vi "FABR-Init I-O Plot.vi"(0 "I-O":refnum<vi>, 5 "IOLegend":refnum<vi>, 7 "Freq":dbl[](array[numeric]), 9 "Level":dbl[](array[numeric]), 11 "error in (no error)":errorcluster) -> (15 "error out":errorcluster)   [LabVIEW 2020]
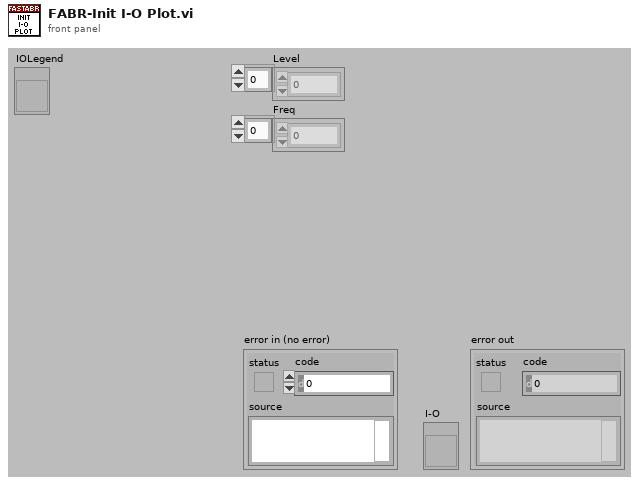
[diagram p1: front panel]
types:
  T1 = enum16{"User", "Prism", "Kelly", "Dark2", "Sequential", "Hue"}
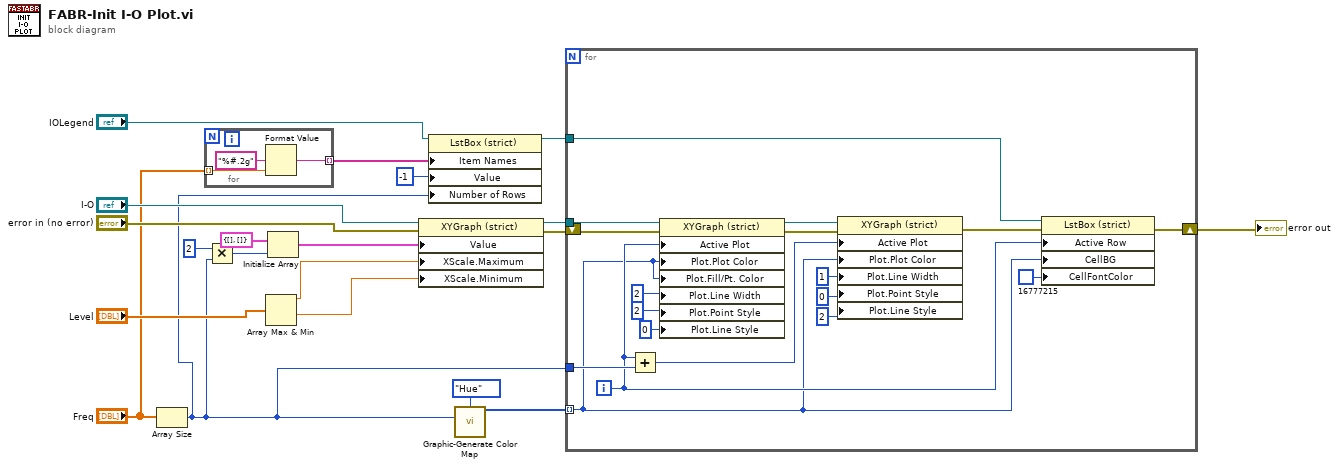
[diagram p0: block diagram]
diagram:
  n1 = Array Size(array="Freq") -> (size(s)=w1:i32)
  n2 = for {
    tunnel: "Freq" -> [w23] mode=indexing
    tunnel: [w21] -> w4 mode=indexing
    n3 = Format Value(format string="%#.2g", value (0)=w23) -> (output string=w21:string)  [unwired: 1 in]
  }
  n4 = Multiply(x=2, y=w1) -> (x*y=w12:i32)
  n5 = Array Max & Min(array="Level") -> (max value=w18:dbl, min value=w17:dbl)  [unwired: 2 out]
  n6 = Initialize Array(cluster{dbl[], dbl[]} {[], []}, w12) -> (w11:cluster{dbl[], dbl[]}[])
  n7 = property class="XYGraph (strict)"(reference="I-O", error in="error in (no error)", "Value"=w11, "XScale.Maximum"=w18, "XScale.Minimum"=w17) -> (reference out=w10:refnum<vi>, error out=w9:errorcluster)
  n8 = property class="LstBox (strict)"(reference="IOLegend", "Item Names"=w4, "Value"=-1 ("Focus Row"), "Number of Rows"=w1) -> (reference out=w3:refnum<vi>)  [unwired: 1 in, 1 out]
  n9 = call "Graphic-Generate Color Map.vi"("Map"=T1."Hue", "Size"=w1) -> ("Colors"=w8:u32[])  [unwired: 13 in]
  n10 = for {
    tunnel: w10 -> [w41]
    tunnel: w8 -> [w25] mode=indexing
    tunnel: w1 -> [w35]
    shift-right: [w27] -> w7
    shift-left: w9 -> [w40]
    tunnel: w3 -> [w29]
    i -> [w26]
    n11 = Add(x=w26, y=w35) -> (x+y=w34:i32)
    n12 = property class="XYGraph (strict)"(reference=w41, error in=w40, "Active Plot"=w26, "Plot.Plot Color"=w25, "Plot.Fill/Pt. Color"=w25, "Plot.Line Width"=u8 2, "Plot.Point Style"=u8 2, "Plot.Line Style"=u8 0) -> (reference out=w37:refnum<vi>, error out=w36:errorcluster)
    n13 = property class="XYGraph (strict)"(reference=w37, error in=w36, "Active Plot"=w34, "Plot.Plot Color"=w25, "Plot.Line Width"=u8 1, "Plot.Point Style"=u8 0, "Plot.Line Style"=u8 2) -> (error out=w28:errorcluster)  [unwired: 1 out]
    n14 = property class="LstBox (strict)"(reference=w29, error in=w28, "Active Row"=w26, "CellBG"=w25, "CellFontColor"=u32 16777215) -> (error out=w27:errorcluster)  [unwired: 1 out]
  }
  "error out" <- w7
